vi "Configure Generator Power.vi"(8 "error in (no error)":errorcluster, 10 "power, dBm":dbl=-25.0, 11 "Arinst SSA-TG in":refnum<class "PL Arinst SSA-TG.lvclass">) -> (0 "error out":errorcluster, 3 "Arinst SSA-TG out":refnum<class "PL Arinst SSA-TG.lvclass">)   [LabVIEW 2015, in "PL Arinst SSA-TG.lvclass"]
doc: "Configures generator power."
uses:
  PL Arinst SSA-TG.lvclass
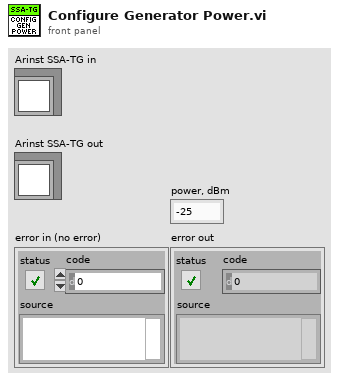
[diagram p1: front panel]
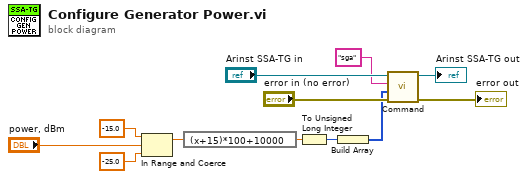
[diagram p0: block diagram]
diagram:
  n1 = In Range and Coerce(upper limit=-15.0, x="power, dBm", lower limit=-25.0) -> (coerced(x)=w6:dbl)  [unwired: 1 out]
  n2 = expression code="(x+15)*100+10000"(w6) -> (w2:dbl)
  n3 = To Unsigned Long Integer(number=w2) -> (unsigned 32bit integer=w1:u32)
  n4 = Build Array(w1) -> (w7:u32[])
  n5 = call "Command.vi"("error in (no error)"="error in (no error)", "arguments (none)"=w7, "command"="sga", "Arinst SSA-TG in"="Arinst SSA-TG in") -> ("error out"=→"error out":errorcluster, "Arinst SSA-TG out"=→"Arinst SSA-TG out":refnum<class "PL Arinst SSA-TG.lvclass">)  [unwired: 5 in, 1 out]
